vi "Actor Core.vi"(8 "error in":errorcluster, 11 "Channel in":refnum<class "Channel.lvclass">) -> (0 "error out":errorcluster, 3 "Actor out":refnum<class "Actor.lvclass">)   [LabVIEW 2015, in "Channel.lvlib" / "Channel.lvclass"]
doc: "(<B>Filename</B>: Actor Framework.lvlib:Actor.lvclass:Actor Core.vi)\n\nReceives messages to the actor, reacts to them, and initiates any error handling that may shut the actor down.\n\nDescendant classes may override this VI to append parallel tasks for the actor to complete while it handles messages. Overrides use the Call Parent Method node."
uses:
  Channel.lvclass
  <vilib>/ActorFramework/Actor/Actor.lvclass
  Channel.lvclass/Channel.ctl
  <userlib>/_Win8uiFramework/ViewableActor.lvclass
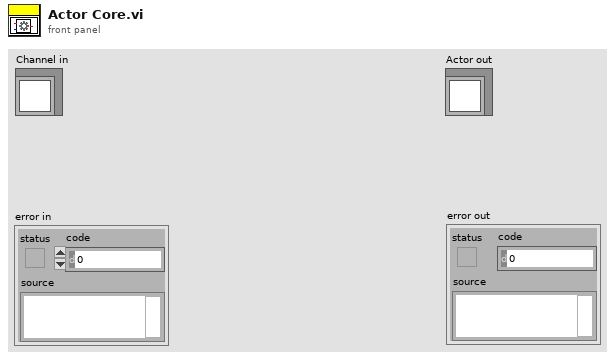
[diagram p1: front panel]
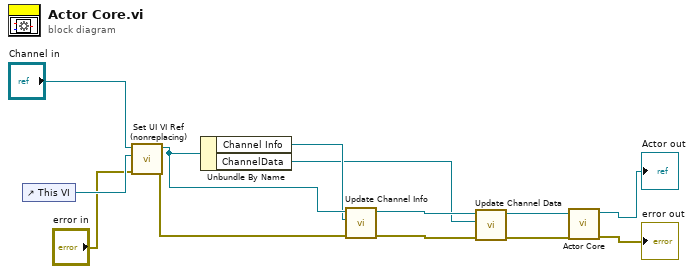
[diagram p0: block diagram]
diagram:
  n1 = control-ref of="This VI"() -> (w10:refnum<vi>)
  n2 = call <userlib>:"Set UI VI Ref (nonreplacing).vi"("error in (no error)"="error in", "UI VI Ref"=w10, "ViewableActor in"="Channel in") -> ("error out"=w8:errorcluster, "ViewableActor out"=w7:refnum<class "Channel.lvclass">)  [unwired: 6 in, 1 out]
  n3 = Unbundle By Name(w7) -> ("Channel Info"=w6:refnum<class "ChannelInfo.lvclass">, "ChannelData"=w1:refnum<class "ChannelData.lvclass">)
  n4 = call "Update Channel Info.vi"("error in (no error)"=w8, "Channel Info"=w6, "Channel in"=w7) -> ("error out"=w4:errorcluster, "Channel out"=w5:refnum<class "Channel.lvclass">)  [unwired: 7 in]
  n5 = call "Update Channel Data.vi"("error in (no error)"=w4, "ChannelData"=w1, "Channel in"=w5) -> ("error out"=w2:errorcluster, "Channel out"=w3:refnum<class "Channel.lvclass">)  [unwired: 7 in]
  n6 = call-parent "Actor Core.vi"("error in"=w2, "Actor in"=w3) -> ("error out"=→"error out":errorcluster, "Actor out"=→"Actor out":refnum<class "Actor.lvclass">)  [unwired: 8 in]
